vi "MainLoop2.vi"() -> ()   [LabVIEW 2021] (continued)
                                                                                                                                                                                                                                                                                                                                                                                                                                                                                                                                                                                                                                                                                                                                                                                                                                                                                                                                                                                                                                                                                                                                                                                                                                                                                                                                                                                                                                                                                                                                                                                                                                                                                                                                                                                                                                                                                                                                                                                                                                                                                                                                                                                                                                                                                                                                                                                                                                                                                                                                                                                                                                                                                                                                                                                                                                                                                                                                                                                                                                                                                                                                                                                                                                                                                                                                                                                                                                                                                                                                                                                                                                                                                                                                                                                                                                                                                                                                                                                                                                                                                                                                                                                                                                                                                                                                                                                                                                                                                                                                                                                                                                                                                                                                                                                                                                                                                                                                                                                                                                                                                                                                                                                                                                                                                                                                                                                                                                                                                                                                                                                                                                                                                                                                                                                                                                                                                                                                                                                                                                                                                                                                                                                                                                                                                                                                                                                                                                                                                                                                                                                                                                                                                                                                                                                                                                                                                                                                                                                                                                                                                                                                                                                                                                                                                                                                                                                                                                                                                                                                                                                                                                                                                                                                                                                                                                                                                                                                                                                                                                                                                                                                                                                                                                                                                                                                                                                                                                                                                                                                                                                                                                                                                                                                                                                                                                                                                                                                                                                                                                                                                                                                                                                                                                                                                                                                                                                                                                                                                                                                                                                                                                                                                                                                                                                                                                                                                                                                                                                                                                                                                                                                                                                                                                                                                                                                                                                                                                                                                                                                                                                                                                                                                                                                                                                                                                                                                                                                                                                                                                                                                                                                                                                                                                                                                                                                                                                                                                                                                                                                                                                                                                                                                                                                                                                                                                                                                                                                                                                                                                                                                                                                                                                                                                                                                                                                                                                                                                                                                                                                                                                                                                                                                                                                                                                                                                                                                                                                                                                                                                                                                                                                                                                                                                                                                                                                                                                                                                                                                                                                                                                                                                                                                                                                                                                                                                                                                                                                                                                                                                                                                                                                                                                                                                                                                                                                                                                                                                                                                                                                                                                                                                                                                                                                                                                                                                                                                                                                                                                                                                                                                                                                                                                                                                                                                                                                                                                                                                                                                                                                                                                                                                                                                                                                                                                                                                                                                                                                                                                                                                                                                                                                                                                                                                                                                                                                                                                                                                                                                                                                                                                                                                                                                                                                                                                                                                                                                                                                                                                                                                                                                                                                                                                                                                                                                                                                                                                                                                                                                                                                                                                                                                                                                                                                                                                                                                                                                                                                                                                                                                                                                                                                                                                                                                                                                                                                                                                                                                                                                                                                                                                                                                                                 256670997", "DINNER TIME", "0", "120", "0", "0", "0"], ["15/06/2022", "17:53:34", "256672767", "1 pellets delivered total", "0", "120", "0", "0", "0"], ["15/06/2022", "17:53:34", "256673260", "1 pellets delivered total", "0", "120", "1", "0", "0"], ["15/06/2022", "17:53:47", "256686605", "MIDDLE BEAM BREAK", "0", "201", "0", "0", "0"], ["15/06/2022", "17:53:48", "256686629", "Condition: m - 201", "0", "201", "0", "0", "0"], ["15/06/2022", "17:53:49", "256688396", "Nest beam break", "0", "201", "0", "0", "0"], ["15/06/2022", "17:53:53", "256692528", "4127 ms in nest", "0", "201", "0", "0", "0"], ["15/06/2022", "17:53:53", "256692552", "Nest beam break", "0", "201", "0", "0", "0"], ["15/06/2022", "17:53:56", "256694657", "SOCIAL TIME", "0", "201", "0", "0", "0"], ["15/06/2022", "17:53:59", "256697678", "SOCIAL TIME", "0", "201", "0", "0", "3009"], ["15/06/2022", "17:53:59", "256697702", "3009 ms social time", "0", "201", "0", "0", "3009"], ["15/06/2022", "17:54:00", "256699281", "MIDDLE BEAM BREAK", "0", "201", "0", "0", "0"], ["15/06/2022", "17:54:00", "256699306", "Condition: m - 201", "0", "201", "0", "0", "0"], ["15/06/2022", "17:54:05", "256704099", "DINNER TIME", "0", "201", "0", "0", "0"], ["15/06/2022", "17:54:06", "                                                                                                                                                                                                                                                                                                                                                                                                                                                                                                                                                                                                                                                                                                                                                                                                                                                                                                                                                                                                                                                              256705543", "Inter-pellet_interval", "0", "201", "0", "0", "0"], ["15/06/2022", "17:54:17", "                                                                                                                                                                                                                                                                                                                                                                                                                                                                                                                                                                                                                                                                                                                                                                                                                                                                                                                                                                                                                                                                                                                                                                                                                                                                                                                                                                                                                                                                                                                                                                                                                                                                                                                                                                                                                                                                                                                                                                                                                                                                                                                                                                                                                                                                                                                                                                                                                                                                                                                                                                                                                                                                                                                                                                                                                                                                                                                                                                                                                                                                                                                                                                                                                                                                                                                                                                                                                                                                                                                                                                                                                                                                                                                                                                                                                                                                                                                                                                                                                                                                                                                                                                                                                                                                                                                                                                                                                                                                                                                                                                                                                                                                                                                                                                                                                                                                                                                                                                                                                                                                                                                                                                                                                                                                                                                                                                                                                                                                                                                                                                                                                                                                                                                                                                                                                                                                                                                                                                                                                                                                                                                                                                                                                                                                                                                                                                                                                                                                                                                                                                                                                                                                                                                                                                                                                                                                                                                                                                                                                                                                                                                                                                                                                                                                                                                                                                                                                                                                                                                                                                                                                                                                                                                                                                                                                                                                                                                                                                                                                                                                                                                                                                                                                                                                                                                                                                                                                                                                                                                                                                                                                                                                                                                                                                                                                                                                                                                                                                                                                                                                                                                                                                                                                                                                                                                                                                                                                                                                                                                                                                                                                                                                                                                                                                                                                                                                                                                                                                                                                                                                                                                                                                                                                                                                                                                                                                                                                                                                                                                                                                                                                                                                                                                                                                                                                                                                                                                                                                                                                                                                                                                                                                                                                                                                                                                                                                                                                                                                                                                                                                                                                                          256715699", "3 pellets delivered total", "0", "201", "0", "0", "0"], ["15/06/2022", "17:54:17", "                                                                                                                                                                                                                                                                                                                                                                                                                                                                                                                                                                                                                                                                                                                                                                                                                                                                                                                                                                                                                                                                                                                                                                                                                                                                                                                                                                                                                                                                                                                                                                                                                                                                                                                                                                                                                                                                                                                                                                                                                                                                                                                                                                                                                                                                                                                                                                                                                                                                                                                                                                                                                                                                                                                                                                                                                                                                                                                                                                                                                                                                                                                                                                                                                                                                                                                                                                                                                                                                                                                                                                                                                                                                                                                                                                                                                                                                                                                                                                                                                                                                                                                                                                                                                                                                                                                                                                                                                                                                                                                                                                                                                                                                                                                                                                                                                                                                                                                                                                                                                                                                                                                                                                                                                                                                                                                                                                                                                                                                                                                                                                                                                                                                                                                                                                                                                                                                                                                                                                                                                                                                                                                                                                                                                                                                                                                                                                                                                                                                                                                                                                                                                                                                                                                                                                                                                                                                                                                                                                                                                                                                                                                                                                                                                                                                                                                                                                                                                                                                                                                                                                                                                                                                                                                                                                                                                                                                                                                                                                                                                                                                                                                                                                                                                                                                                                                                                                                                                                                                                                                                                                                                                                                                                                                                                                                                                                                                                                                                                                                                                                                                                                                                                                                                                                                                                                                                                                                                                                                                                                                                                                                                                                                                                                                                                                                                                                                                                                                                                                                                                                                                                                                                                                                                                                                                                                                                                                                                                                                                                                                                                                                                                                                                                                                                                                                                                                                                                                                                                                                                                                                                                                                                                                                                                                                                                                                                                                                                                                                                                                                                                                                                                                                                                                                                                                                                                                                                                                                                                                                                                                                                                                                              256716167", "3 pellets delivered total", "0", "201", "3", "0", "0"], ["15/06/2022", "17:54:50", "256749394", "3 pellets delivered total", "0", "120", "0", "0", "0"], ["15/06/2022", "17:54:50", "256749419", "Condition: j - 120", "0", "120", "0", "0", "0"], ["15/06/2022", "17:54:52", "256750710", "Nest beam break", "0", "120", "0", "0", "0"], ["15/06/2022", "18:19:22", "                                                                                                                                                                                                                                                                                                                                                                                                                                                                                                                                                                                                                                                                                                                                                                                                                                                                                                                                                                                                                                                                                                                                                                                                                                                                                                                                                                                                                                                                                                                                                                                                                                                                                                                                                                                                                                                                                                                                                                                                                                                                                                                                                                                                                                                                                                                                                                                                                                                                                                                                                                                                                                                                                                                                                                                                                                                                                                                                                                                                                                                                                                                                                                                                                                                                                                                                                                                                                                                                                                                                                                                                                                                                                                                                                                                                                                                                                                                                                                                                                                                                                                                                                                                                                                                                                                                                                                                                                                                                                                                                                                                                                                                                                                                                                                                                                                                                                                                                                                                                                                                                                                                                                                                                                                                                                                                                                                                                                                                                                                                                                                                                                                                                                                                                                                                                                                                                                                                                                                                                                                                                                                                                                                                                                                                                                                                                                                                                                                                                                                                                                                                                                                                                                                                                                                                                                                                                                                                                                                                                                                                                                                                                                                                                                                                                                                                                                                                                                                                                                                                                                                                                                                                                                                                                                                                                                                                                                                                                                                                                                                                                                                                                                                                                                                                                                                                                                                                                                                                                                                                                                                                                                                                                                                                                                                                                                                                                                                                                                                                                                                                                                                                                                                                                                                                                                                                                                                                                                                                                                                                                                                                                                                                                                                                                                                                                                                                                                                                                                                                              258221447", "1469059 ms in nest", "1469059", "120", "0", "0", "0"]]
  in  "Save event file?":bool=TRUE
  in  "file path (dialog if empty)":path=path "C:/Data/av_maze/cohort1/mouseX_202206XXtxt"
  # "Social\n\nWater\n\nFood\n\nMiddle 1\n\nMiddle 2\n\nHome cage"
  # "Low (0)     Medium (1)    High(2)"
  # "Pellets \n\nWater drops\n\nSocial time (ms)"
  # "This should stay at 1"
  # "Social                Water                  Food               Middle            Middle 2       Home cage"
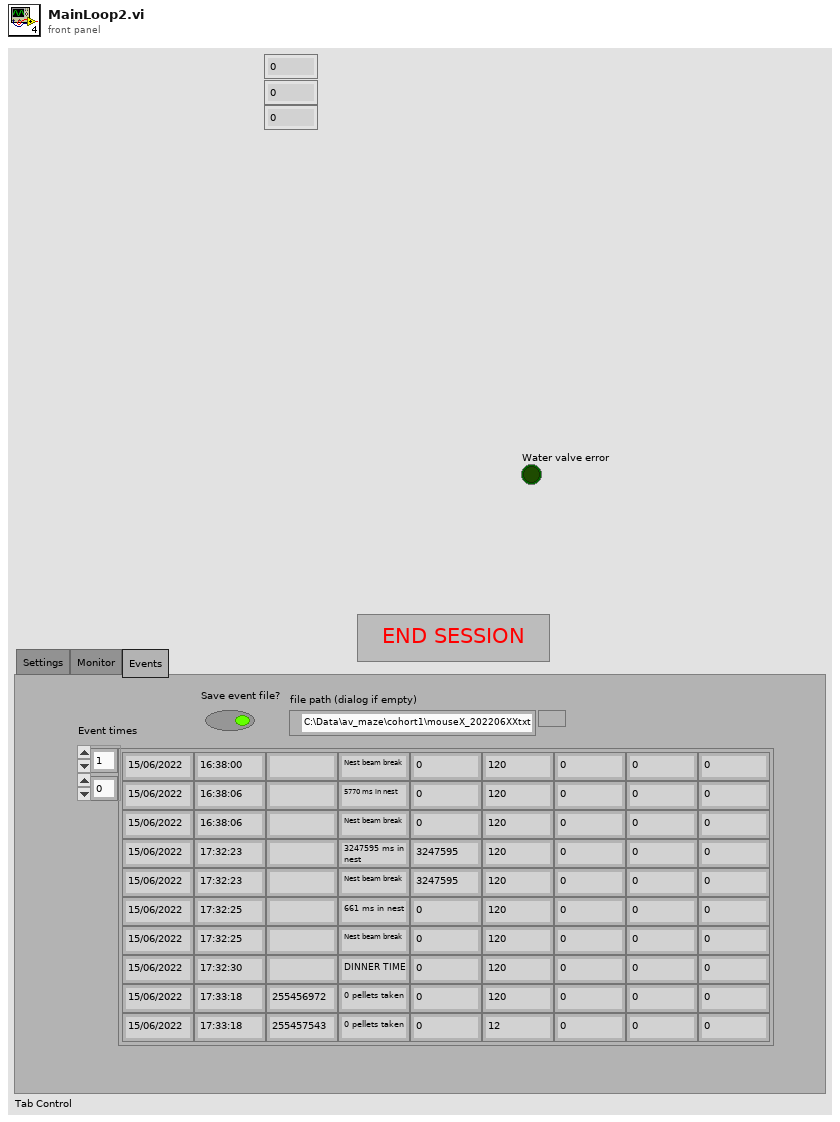
[diagram p1: front panel]
types:
  T1 = enum32{"All drives change and different", "One drive changes", "All drives same, but change"}
  T2 = typedef "XDNodeRunTimeDep.lvlib/timing_clust.ctl" = cluster{"Expected End [f-1]":u64, "Actual End [f-1]":u64, "Finished Late? [f-1]":bool, "Expected End [i-1]":u64, "Actual End [i-1]":u64, "Finished Late? [i-1]":bool, "Expected Start [i]":u64, "Actual Start [i]":u64, "Expected Start [f]":u64, "Actual Start [f]":u64, "Source Name":string, "Structure Name":string, "Period":i64, "Deadline":i64, "Offset":i64, "Start":i64, "Priority":i32, "Timeout":i32, "Mode":T3, "Wakeup Reason":T4, "Error":errorcluster, "Source Type":string, "Secondary Source Type":string, "Global End Time":u64, "Global Start Time":u64, "Frame Duration":u64, "Iteration Duration":u64, "Assigned CPU":i32, "I/O Scan Engine Mode":u32}
  T3 = typedef "XDNodeRunTimeDep.lvlib/nitl_modes.ctl" = enum32{"No Change", "Process missed periods, maintain original phase", "Discard missed periods, maintain original phase", "Process missed periods, ignore original phase", "Discard missed periods, ignore original phase"}
  T4 = typedef "XDNodeRunTimeDep.lvlib/wakeup.ctl" = enum32{"Normal", "Aborted", "Asynchronous wakeup", "Timing source error", "Timed loop error", "Timeout"}
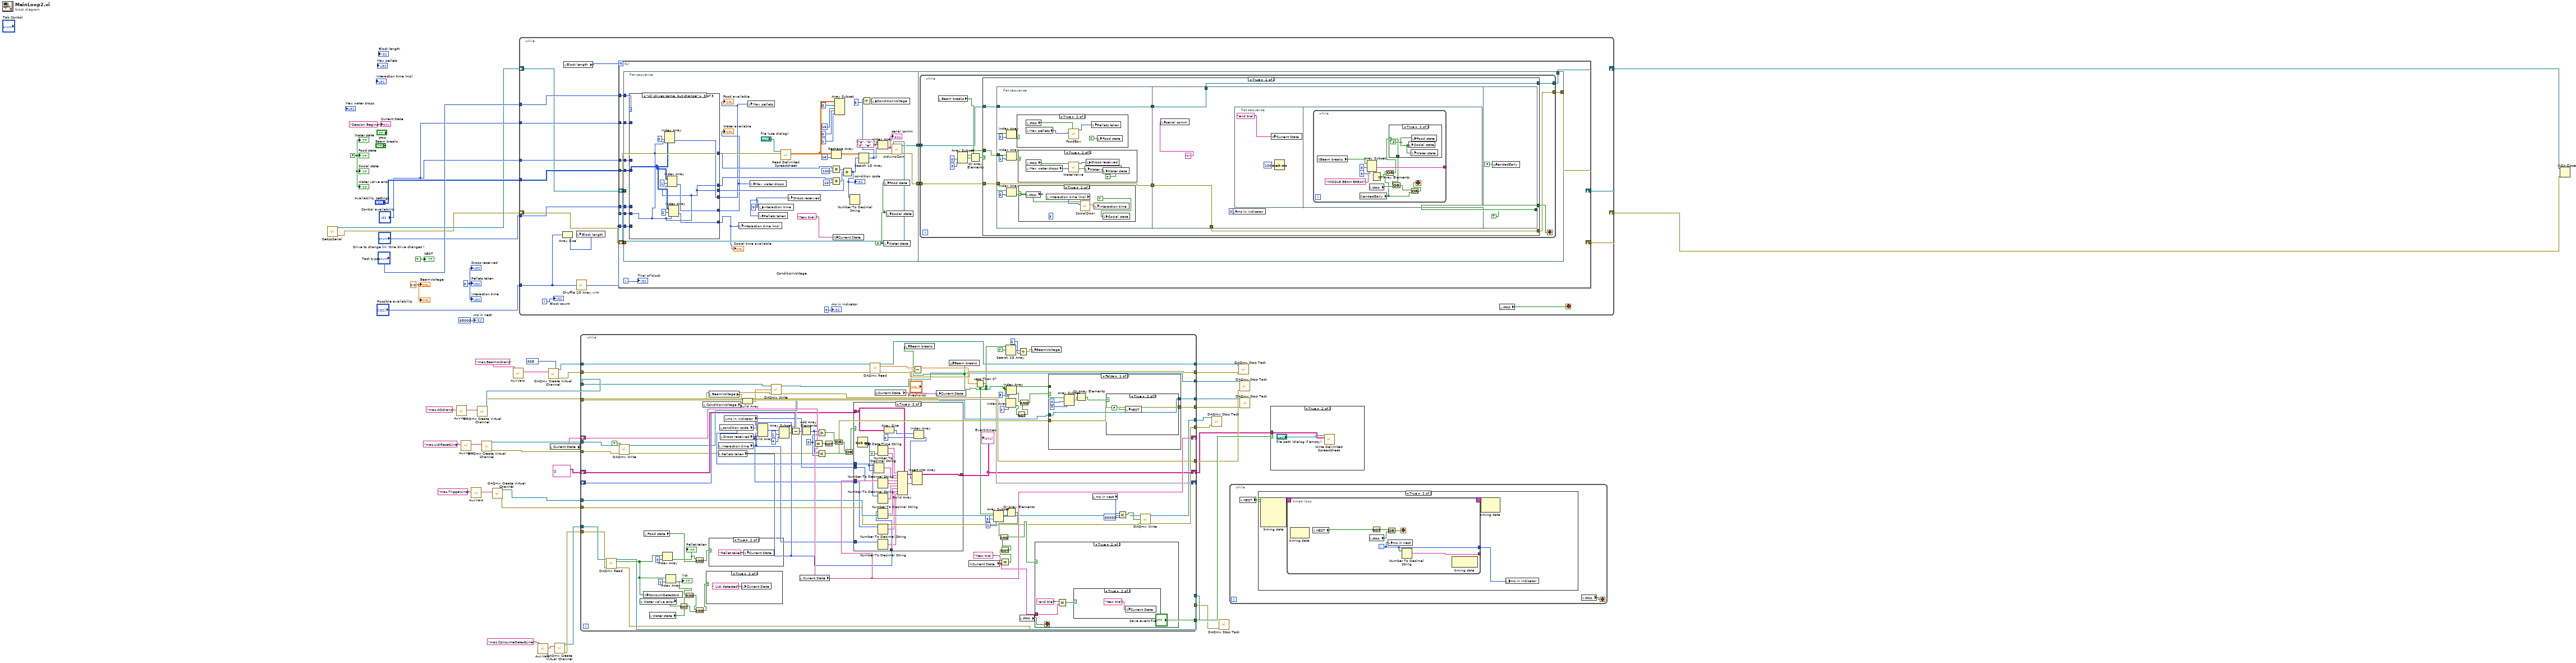
[diagram p0: block diagram]
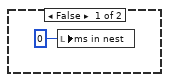
[diagram p2: hidden frame]
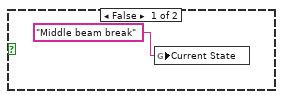
[diagram p7: hidden frame]
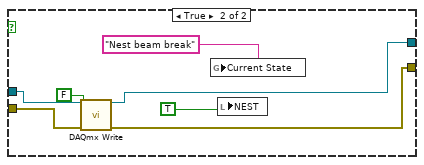
[diagram p9: hidden frame]
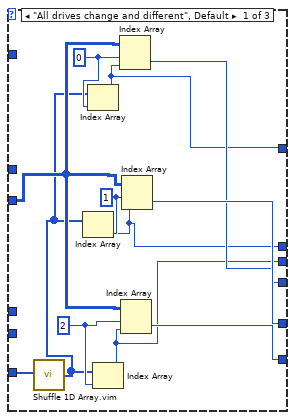
[diagram p11: hidden frame]
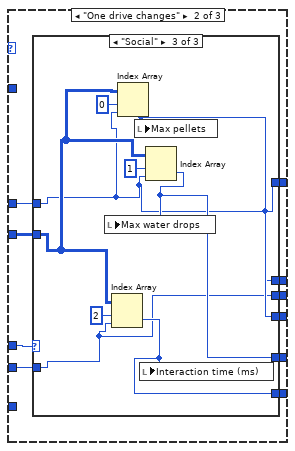
[diagram p12: hidden frame]
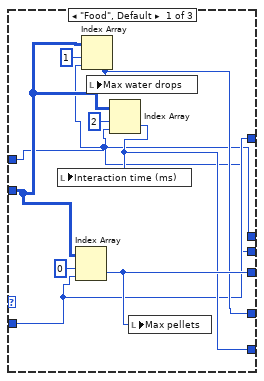
[diagram p13: hidden frame]
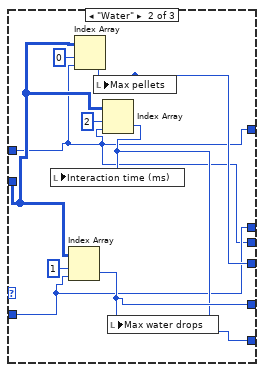
[diagram p14: hidden frame]
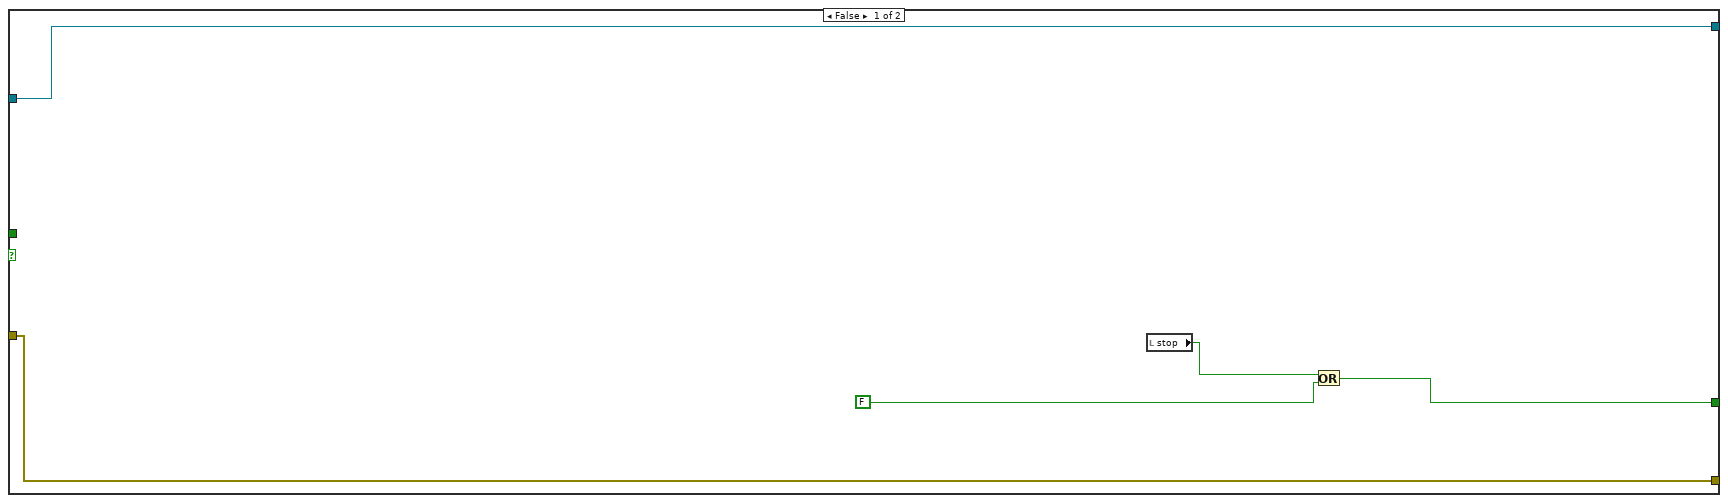
[diagram p15: hidden frame]
diagram:
  w13 = FALSE ("Water state")
  w22 = u32 0 ("Pellets taken")
  w33 = 0.0 ("BeamVoltage")
  w38 = 10083 items=["Default"=-1, "RSE"=10083, "NRSE"=10078, "Differential"=10106, "Pseudodifferential"=12529] ("input terminal configuration")
  n1 = call "SetUpSerial.vi"() -> ("error out"=w25:errorcluster, "VISA resource name out"=w40:refnum<visa-resource-name>)  [unwired: 10 in]
  n2 = call "AuxVars.vi"("key"="maz.AOchans") -> ("value"=w29:string)  [unwired: 9 in, 1 out]
  n3 = call "AuxVars.vi"("key"="maz.LickResetLine") -> ("value"=w12:string)  [unwired: 9 in, 1 out]
  n4 = call "AuxVars.vi"("key"="maz.TriggerLine") -> ("value"=w6:string)  [unwired: 9 in, 1 out]
  n5 = call-poly <vilib>:"DAQmx Create Virtual Channel.vi"("physical channels"=w29) -> ("task out"=w35:refnum<k21>, "error out"=w34:errorcluster)  [unwired: 13 in]
  n6 = call-poly <vilib>:"DAQmx Create Virtual Channel.vi"("lines"=w12) -> ("task out"=w10:refnum<k21>, "error out"=w9:errorcluster)  [unwired: 13 in]
  n7 = call-poly <vilib>:"DAQmx Create Virtual Channel.vi"("lines"=w6) -> ("task out"=w4:refnum<k21>, "error out"=w3:errorcluster)  [unwired: 13 in]
  n8 = call "AuxVars.vi"("key"="maz.BeamAIchans") -> ("value"=w27:string)  [unwired: 9 in, 1 out]
  n9 = while {
    tunnel: "Task type" -> [w66]
    tunnel: "Drive to change (in 'One drive changes')" -> [w65]
    tunnel: "Possible availability" -> [w60]
    tunnel: "Availability settings" -> [w64]
    tunnel: "Control availability" -> [w63]
    tunnel: "Control availability" -> [w62]
    shift-right: [w53] -> w26
    shift-left: w40 -> [w55]
    shift-right: [w52] -> w39
    shift-left: w25 -> [w54]
    i -> [w58]
    stop <- w56 stop-if-true
    n10 = Array Size(array=w60) -> (size(s)=w59:i32)
    n11 = local read "Block length"() -> (w61:i32)
    n12 = local write "Block length"(w59) -> ()
    n13 = call "Shuffle 1D Array.vim"("array"=w60) -> ("shuffled array"=w57:i32[])  [unwired: 4 in]
    n14 = for {
      N: w61 -> [_]
      tunnel: w66 -> [w80]
      tunnel: w65 -> [w79]
      tunnel: w57 -> [w78] mode=indexing
      tunnel: w64 -> [w77]
      tunnel: w63 -> [w76]
      tunnel: w62 -> [w75]
      tunnel: w57 -> [w73]
      shift-right: [w68] -> w53
      shift-left: w55 -> [w72]
      shift-right: [w67] -> w52
      shift-left: w54 -> [w71]
      i -> [w74]
      n15 = flat-sequence {
        tunnel: w80 -> [w118]
        tunnel: w79 -> [w117]
        tunnel: w78 -> [w116]
        tunnel: w77 -> [w115]
        tunnel: w76 -> [w114]
        tunnel: w75 -> [w113]
        tunnel: w73 -> [w112]
        tunnel: w72 -> [w93]
        tunnel: w71 -> [w92]
        tunnel: [w82] -> w70
        tunnel: [w81] -> w69
        tunnel: w70 -> [w179]
        tunnel: w69 -> [w178]
        tunnel: [w177] -> w68
        tunnel: [w176] -> w67
        frame #0 {
          w84 = FALSE ("Social state")
          w85 = u32 0 ("interaction time")
          n16 = case shown="\"All drives same, but change\"" w118 {
            tunnel: w117 -> [_ w140 _]
            tunnel: w116 -> [_ w139 w168]
            tunnel: w115 -> [w130 w138 w172]
            tunnel: w114 -> [_ _ _]
            tunnel: w113 -> [_ w137 _]
            tunnel: [w122 w136 w171] -> w90
            tunnel: [w123 w135 w170] -> w89
            tunnel: [w127 w134 w169] -> w91
            tunnel: w112 -> [w129 _ _]
            tunnel: [w121 w133 w168] -> w109
            tunnel: [w120 w132 w168] -> w108
            tunnel: [w119 w131 w168] -> w107
            frame "All drives change and different", Default {
              w126 = 0 ("index")
              w125 = 1 ("index")
              w128 = 2 ("index")
              n17 = call "Shuffle 1D Array.vim"("array"=w129) -> ("shuffled array"=w124:i32[])  [unwired: 4 in]
              n18 = Index Array(array=w124, index=w125) -> (element=w120:i32)
              n19 = Index Array(array=w124, index=w126) -> (element=w121:i32)
              n20 = Index Array(array=w124, index=w128) -> (element=w119:i32)
              n21 = Index Array(array=w130, index (row)=w126, index (col)=w121) -> (element=w122:i32)
              n22 = Index Array(array=w130, index (row)=w128, index (col)=w119) -> (element=w127:i32)
              n23 = Index Array(array=w130, index (row)=w125, index (col)=w120) -> (element=w123:i32)
            }
            frame "One drive changes" {
              n24 = case shown="\"Social\"" w140 {
                tunnel: w139 -> [w142 w151 w159]
                tunnel: w138 -> [w146 w155 w164]
                tunnel: w137 -> [w141 w150 w160]
                tunnel: [w145 w154 w161] -> w136
                tunnel: [w144 w153 w163] -> w135
                tunnel: [w143 w152 w162] -> w134
                tunnel: [w142 w150 w160] -> w133
                tunnel: [w141 w151 w160] -> w132
                tunnel: [w141 w150 w159] -> w131
                frame "Food", Default {
                  n25 = Index Array(array=w146, index (row)=0 ("index"), index (col)=w142) -> (element=w145:i32)
                  n26 = Index Array(array=w146, index (row)=1, index (col)=w141) -> (element=w144:i32)
                  n27 = local write "Max water drops"(w144) -> ()
                  n28 = Index Array(array=w146, index (row)=2 ("disabled index (row)"), index (col)=w141) -> (element=w143:i32)
                  n29 = local write "Interaction time (ms)"(w143) -> ()
                  n30 = local write "Max pellets"(w145) -> ()
                }
                frame "Water" {
                  n31 = Index Array(array=w155, index (row)=1 ("index"), index (col)=w151) -> (element=w153:i32)
                  n32 = Index Array(array=w155, index (row)=0, index (col)=w150) -> (element=w154:i32)
                  n33 = local write "Max pellets"(w154) -> ()
                  n34 = Index Array(array=w155, index (row)=2 ("disabled index (row)"), index (col)=w150) -> (element=w152:i32)
                  n35 = local write "Interaction time (ms)"(w152) -> ()
                  n36 = local write "Max water drops"(w153) -> ()
                }
                frame "Social" {
                  n37 = Index Array(array=w164, index (row)=2 ("index"), index (col)=w159) -> (element=w162:i32)
                  n38 = Index Array(array=w164, index (row)=0, index (col)=w160) -> (element=w161:i32)
                  n39 = local write "Max pellets"(w161) -> ()
                  n40 = local write "Interaction time (ms)"(w162) -> ()
                  n41 = Index Array(array=w164, index (row)=1 ("disabled index (row)"), index (col)=w160) -> (element=w163:i32)
                  n42 = local write "Max water drops"(w163) -> ()
                }
              }
            }
            frame "All drives same, but change" {
              n43 = Index Array(array=w172, index (row)=0, index (col)=w168) -> (element=w171:i32)
              n44 = Index Array(array=w172, index (row)=1, index (col)=w168) -> (element=w170:i32)
              n45 = Index Array(array=w172, index (row)=2, index (col)=w168) -> (element=w169:i32)
            }
          }
          "Food available" <- w90
          "Water available" <- w89
          "Social time available" <- w91
          n46 = local write "Interaction time (ms)"(w91) -> ()
          n47 = local write "Max pellets"(w90) -> ()
          n48 = local write "Max water drops"(w89) -> ()
          n49 = local write "interaction time"(w85) -> ()
          n50 = local write "Pellets taken"(w85) -> ()
          n51 = call-poly <vilib>:"Read Delimited Spreadsheet.vi"("file path (dialog if empty)"="file (use dialog)") -> ("all rows"=w99:dbl[][])  [unwired: 9 in, 5 out]
          n52 = local write "Drops received"(w85) -> ()
          n53 = Reshape Array(w99, 16 ("dimension size")) -> (w98:dbl[])
          n54 = Multiply(x=w109, y=100) -> (x*y=w105:i32)
          n55 = Multiply(x=w108, y=10) -> (x*y=w106:i32)
          n56 = global write "GlobalSTATE.vi" "Current State"("New trial " ("string")) -> ()
          n57 = Array Subset(array=w99, index (row)=0 ("index"), length (row)=16 ("length"), index (col)=0 ("index"), length (col)=1 ("length")) -> ()  [unwired: 1 out]
          n58 = Compound Arithmetic op=ADD(w105, w106, w107) -> (w94:i32)
          "condition code" <- w94
          n59 = Number To Decimal String(number=w94) -> ()  [unwired: 1 in, 1 out]
          n60 = Search 1D Array(1D array=w98, element=w94) -> (index of element=w87:i32)  [unwired: 1 in]
          n61 = Divide(x=w87, y=5) -> (x/y=w88:dbl)
          n62 = local write "ConditionVoltage"(w88) -> ()
          n63 = Index Array(array=string[] ["a", "b", "c", "d", "e", "f", "g", "h", "i", "j", "k", "l", "m", "n", "o"], index=w87) -> (element=w95:string)
          "serial comm" <- w95
          n64 = local write "Water state"(w84) -> ()
          n65 = local write "Food state"(w84) -> ()
          n66 = local write "Social state"(w84) -> ()
          n67 = call "ArduinoCom.vi"("error out"=w92, "write buffer"=w95, "VISA resource name out"=w93) -> ("error out 2"=w81:errorcluster, "VISA resource name out 2"=w82:refnum<visa-resource-name>)  [unwired: 7 in]
        }
        frame #1 {
          n68 = while {
            tunnel: w179 -> [w183]
            tunnel: w178 -> [w182]
            tunnel: [w181] -> w177
            tunnel: [w180] -> w176
            stop <- w184 stop-if-true
            n69 = local read "Beam breaks"() -> (w185:bool[])
            n70 = Array Subset(array=w185, index=0, length=3) -> (w188:bool[])
            n71 = Or Array Elements(Boolean array=w188) -> (logical OR=w189:bool)
            n72 = case shown="True" w189 {
              tunnel: w185 -> [_ w202]
              tunnel: [w192 w201] -> w184
              tunnel: w183 -> [w191 w199]
              tunnel: w182 -> [w190 w197]
              tunnel: [w191 w196] -> w181
              tunnel: [w190 w195] -> w180
              frame False {
                n73 = local read "stop"() -> (w193:bool)
                n74 = Or(x=w193, y=FALSE ("stop")) -> (x .or. y?=w192:bool)
              }
              frame True {
                n75 = flat-sequence {
                  tunnel: w202 -> [w205]
                  tunnel: [w204] -> w200
                  tunnel: w199 -> [w204]
                  tunnel: [w203] -> w198
                  tunnel: w197 -> [w203]
                  tunnel: w200 -> [w227]
                  tunnel: w198 -> [w226]
                  tunnel: [w227] -> w196
                  tunnel: [w226] -> w195
                  tunnel: [TRUE ("stop")] -> w201
                  frame #0 {
                    n76 = Index Array(array=w205, index=2) -> (element=w210:bool)
                    n77 = Index Array(array=w205, index=1) -> (element=w206:bool)
                    n78 = Index Array(array=w205, index=0) -> (element=w208:bool)
                    n79 = case shown="True" w210 {
                      frame False {
                      }
                      frame True {
                        n80 = local read "stop"() -> (w223:bool)
                        n81 = local read "Max pellets"() -> (w224:u32)
                        n82 = call "FoodBox.vi"("STOP"=w223, "Max pellets"=w224) -> ("Pellets taken"=w222:i32)  [unwired: 8 in, 1 out]
                        n83 = local write "Pellets taken"(w222) -> ()
                        n84 = local write "Food state"(TRUE ("Food state")) -> ()
                      }
                    }
                    n85 = case shown="True" w206 {
                      frame False {
                      }
                      frame True {
                        n86 = local read "stop"() -> (w215:bool)
                        n87 = local read "Max water drops"() -> (w216:u32)
                        n88 = call "WaterValve.vi"("Max pulses"=w216, "STOP"=w215) -> ("Error"=w212:bool, "Number pulses"=w214:u32)  [unwired: 8 in]
                        n89 = local write "Water valve error"(w212) -> ()
                        n90 = local write "Drops received"(w214) -> ()
                        n91 = local write "Water state"(TRUE ("Water state")) -> ()
                      }
                    }
                    n92 = case shown="True" w208 {
                      frame False {
                      }
                      frame True {
                        (unwired) 3 ("index")
                        n93 = local read "stop"() -> (w219:bool)
                        n94 = local read "Interaction time (ms)"() -> (w220:u32)
                        n95 = call "SocialDoor.vi"("Interaction time"=w220, "STOP"=w219) -> ("Time spent"=w218:dbl)  [unwired: 9 in]
                        n96 = local write "interaction time"(w218) -> ()
                        n97 = local write "Social state"(TRUE ("Water state")) -> ()
                      }
                    }
                  }
                  frame #1 {
                    n98 = local write "serial comm"("h" ("write buffer")) -> ()
                    n99 = local write "ms in indicator"(0 ("ms in nest")) -> ()
                    n100 = flat-sequence {
                      frame #0 {
                        n101 = global write "GlobalSTATE.vi" "Current State"("end trial " ("string")) -> ()
                        n102 = Wait (ms)(milliseconds to wait=u32 100) -> ()  [unwired: 1 out]
                      }
                      frame #1 {
                        n103 = while {
                          tunnel: ["MIDDLE BEAM BREAK" ("Current State")] -> _
                          stop <- w234 stop-if-true
                          n104 = global read "Global_BeamBreaks.vi" "Beam breaks"() -> (w238:bool[])
                          n105 = global read "EndEarly.vi" "endedEarly"() -> (w232:bool)
                          n106 = Array Subset(array=w238, index=3, length=3) -> (w237:bool[])
                          n107 = local read "stop"() -> (w241:bool)
                          n108 = Or Array Elements(Boolean array=w237) -> (logical OR=w233:bool)
                          n109 = Or(x=w232, y=w233) -> (x .or. y?=w231:bool)
                          n110 = case shown="True" w231 {
                            selector: w231 -> [w243 w244]
                            tunnel: [w243 w244] -> w236
                            frame False {
                            }
                            frame True {
                              w245 = FALSE ("Social state")
                              n111 = local write "Social state"(w245) -> ()
                              n112 = local write "Water state"(w245) -> ()
                              n113 = local write "Food state"(w245) -> ()
                            }
                          }
                          n114 = Or(x=w236, y=w241) -> (x .or. y?=w235:bool)
                          n115 = Or(x=w235, y=w232) -> (x .or. y?=w234:bool)
                        }
                      }
                    }
                  }
                  frame #2 {
                    n116 = global write "EndEarly.vi" "endedEarly"(FALSE ("endedEarly")) -> ()
                  }
                }
              }
            }
          }
        }
      }
      "Trial of block" <- w74
    }
    n117 = local read "stop"() -> (w56:bool)
    "Block count" <- w58
  }
  n118 = call "AuxVars.vi"("key"="maz.ConsumeDetectLine") -> ("value"=w18:string)  [unwired: 9 in, 1 out]
  n119 = call-poly <vilib>:"DAQmx Create Virtual Channel.vi"("input terminal configuration"=w38, "physical channels"=w27) -> ("task out"=w51:refnum<k21>, "error out"=w50:errorcluster)  [unwired: 12 in]
  n120 = local read "Current State"() -> (w41:string)
  n121 = call-poly <vilib>:"DAQmx Create Virtual Channel.vi"("lines"=w18) -> ("task out"=w17:refnum<k21>, "error out"=w16:errorcluster)  [unwired: 13 in]
  n122 = while {
    tunnel: w51 -> [w337]
    tunnel: w50 -> [w336]
    tunnel: [w335] -> w49
    tunnel: [w334] -> w48
    shift-right: [w331] -> _
    shift-left: w41 -> [w330]
    tunnel: ["Save event file?"] -> w37
    tunnel: w35 -> [w323]
    tunnel: w34 -> [w322]
    tunnel: [w314] -> w32
    tunnel: [w313] -> w31
    shift-right: [w307] -> _
    shift-left: _ -> [w312]
    shift-right: [w299] -> w24
    shift-left: string[][] [] -> [w298]
    tunnel: w17 -> [w289]
    tunnel: w16 -> [w288]
    tunnel: [w282] -> w15
    tunnel: [w281] -> w14
    tunnel: w10 -> [w261]
    tunnel: w9 -> [w260]
    tunnel: [w256] -> w8
    tunnel: [w255] -> w7
    tunnel: w4 -> [w251]
    tunnel: w3 -> [w250]
    tunnel: [w249] -> w2
    tunnel: [w248] -> w1
    stop <- w333 stop-if-true
    w304 = u32 0 ("y")
    n123 = call-poly <vilib>:"DAQmx Read.vi"("task/channels in"=w289, "error in"=w288) -> ("task out"=w282:refnum<k21>, "data"=w285:bool[], "error out"=w281:errorcluster)  [unwired: 11 in]
    n124 = call-poly <vilib>:"DAQmx Write.vi"("task/channels in"=w261, "data"=TRUE, "error in"=w260) -> ("task out"=w258:refnum<k21>, "error out"=w257:errorcluster)  [unwired: 10 in, 1 out]
    n125 = local read "Water valve error"() -> (w277:bool)
    n126 = global write "Global_BeamBreaks.vi" "ConsumDetectors"(w285) -> ()
    n127 = local read "Food state"() -> (w278:bool)
    n128 = local read "Water state"() -> (w283:bool)
    n129 = Index Array(array=w285, index=0) -> (element=w279:bool)
    "Pellet taken" <- w279
    n130 = Index Array(array=w285, index=1) -> (element=w284:bool)
    "lick" <- w284
    n131 = Not(x=w277) -> (.not. x?=w276:bool)
    n132 = And(x=w284, y=w283) -> (x .and. y?=w275:bool)
    n133 = And(x=w279, y=w278) -> (x .and. y?=w280:bool)
    n134 = And(x=w275, y=w276) -> (x .and. y?=w274:bool)
    n135 = local read "ConditionVoltage"() -> (w316:dbl)
    n136 = case shown="True" w274 {
      frame False {
      }
      frame True {
        n137 = local write "Current State"(" Lick detected" ("Current State")) -> ()
      }
    }
    n138 = local read "BeamVoltage"() -> (w317:dbl)
    n139 = case shown="True" w280 {
      frame False {
      }
      frame True {
        n140 = local write "Current State"("Pellet taken" ("Current State")) -> ()
      }
    }
    n141 = local read "interaction time"() -> (w293:u32)
    n142 = local read "Pellets taken"() -> (w296:u32)
    n143 = local read "condition code"() -> (w297:i32)
    n144 = local read "Drops received"() -> (w295:u32)
    n145 = local read "ms in indicator"() -> (w294:i32)
    n146 = Build Array(w317, w316) -> (w315:dbl[])
    n147 = Build Array(w294, w297, w296, w295, w293) -> (w300:u32[])
    n148 = call-poly <vilib>:"DAQmx Write.vi"("task/channels in"=w323, "data"=w315, "error in"=w322) -> ("task out"=w314:refnum<k21>, "error out"=w313:errorcluster)  [unwired: 10 in, 1 out]
    n149 = Array Subset(array=w300, index=1, length=4) -> (w307:u32[])
    n150 = Subtract(x=w312, y=w307) -> (x-y=w306:u32[])
    n151 = local read "Current State"() -> (w331:string)
    n152 = Add Array Elements(numeric array=w306) -> (sum=w305:u32)
    n153 = Equal?(x=w330, y=w331) -> (x = y?=w332:bool)
    n154 = Greater?(x=w305, y=w304) -> (0:w310:bool)
    n155 = Less?(x=w305, y=w304) -> (x < y?=w302:bool)
    n156 = Not(x=w332) -> (.not. x?=w311:bool)
    n157 = Or(x=w310, y=w311) -> (x .or. y?=w303:bool)
    n158 = Or(x=w303, y=w302) -> (x .or. y?=w301:bool)
    n159 = case shown="True" w301 {
      tunnel: [w360 w375] -> w299
      tunnel: w331 -> [_ w377]
      tunnel: w298 -> [w360 w374]
      tunnel: w294 -> [_ w370]
      tunnel: w297 -> [_ w368]
      tunnel: w296 -> [_ w366]
      tunnel: w295 -> [_ w364]
      tunnel: w293 -> [_ w361]
      frame False {
      }
      frame True {
        n160 = Tick Count (ms)() -> (millisecond timer value=w381:u32)
        n161 = Number To Decimal String(number=w381, width (-)=w381) -> (decimal integer string=w378:string)
        n162 = Get Date/Time String(want seconds? (F)=TRUE) -> (date string=w380:string, time string=w379:string)  [unwired: 2 in]
        n163 = Number To Decimal String(number=w370) -> (decimal integer string=w369:string)  [unwired: 1 in]
        n164 = Number To Decimal String(number=w368) -> (decimal integer string=w367:string)  [unwired: 1 in]
        n165 = Number To Decimal String(number=w366) -> (decimal integer string=w365:string)  [unwired: 1 in]
        n166 = Number To Decimal String(number=w364) -> (decimal integer string=w363:string)  [unwired: 1 in]
        n167 = Number To Decimal String(number=w361) -> (decimal integer string=w362:string)  [unwired: 1 in]
        n168 = Array Size(array=w374) -> (size(s)=w373:i32[])
        n169 = Build Array(w380, w379, w378, w377, w369, w367, w365, w363, w362) -> (w376:string[])
        n170 = Index Array(array=w373, index=0) -> (element=w371:i32)
        n171 = Insert Into Array(array=w374, index (row)=w371, new element=w376) -> (w375:string[][])  [unwired: 1 in]
      }
    }
    "Event times" <- w299
    n172 = call-poly <vilib>:"DAQmx Read.vi"("task/channels in"=w337, "error in"=w336) -> ("task out"=w335:refnum<k21>, "data"=w327:dbl[], "error out"=w334:errorcluster)  [unwired: 11 in]
    n173 = global read "GlobalSTATE.vi" "Current State"() -> (w329:string)
    n174 = Subtract(x=w327, y="thresholds") -> (x-y=w328:dbl[])
    n175 = local write "Current State"(w329) -> ()
    n176 = global read "GlobalSTATE.vi" "Current State"() -> (w262:string)
    n177 = Less Than 0?(x=w328) -> (x < 0?=w272:bool[])
    n178 = local write "Beam breaks"(w272) -> ()
    n179 = global write "Global_BeamBreaks.vi" "Beam breaks"(w272) -> ()
    n180 = Array Subset(array=w272, index=3, length=2) -> (w290:bool[])
    n181 = Equal?(x="New trial " ("string"), y=w262) -> (x = y?=w266:bool)
    n182 = Not(x=w266) -> (.not. x?=w267:bool)
    n183 = Search 1D Array(1D array=w272, element=TRUE) -> (index of element=w321:i32)  [unwired: 1 in]
    n184 = Index Array(array=w272, index=4) -> (element=w271:bool)
    n185 = Or Array Elements(Boolean array=w290) -> (logical OR=w264:bool)
    n186 = And(x=w264, y=w267) -> (x .and. y?=w263:bool)
    n187 = Index Array(array=w272, index=5) -> (element=w269:bool)
    n188 = Not(x=w271) -> (.not. x?=w270:bool)
    n189 = Divide(x=w321, y=2) -> (x/y=w319:dbl)
    n190 = And(x=w269, y=w270) -> (x .and. y?=w268:bool)
    n191 = local read "stop"() -> (w333:bool)
    n192 = local write "BeamVoltage"(w319) -> ()
    n193 = case shown="True" w263 {
      tunnel: w262 -> [_ w341]
      frame False {
      }
      frame True {
        n194 = Equal?(x="end trial" ("string"), y=w341) -> (x = y?=w340:bool)
        n195 = case shown="True" w340 {
          frame False {
            n196 = global write "GlobalSTATE.vi" "Current State"("Middle beam break" ("Current State")) -> ()
          }
          frame True {
            n197 = global write "GlobalSTATE.vi" "Current State"("New trial" ("Current State")) -> ()
          }
        }
      }
    }
    n198 = case shown="False" w268 {
      tunnel: w272 -> [w351 _]
      tunnel: w258 -> [w346 w357]
      tunnel: w257 -> [w345 w356]
      tunnel: [w346 w354] -> w256
      tunnel: [w345 w353] -> w255
      frame False {
        n199 = Array Subset(array=w351, index=0, length=5) -> (w348:bool[])
        n200 = Or Array Elements(Boolean array=w348) -> (logical OR=w347:bool)
        n201 = case shown="True" w347 {
          frame False {
          }
          frame True {
            n202 = local write "NEST"(FALSE) -> ()
          }
        }
      }
      frame True {
        n203 = call-poly <vilib>:"DAQmx Write.vi"("task/channels in"=w357, "data"=FALSE, "error in"=w356) -> ("task out"=w354:refnum<k21>, "error out"=w353:errorcluster)  [unwired: 10 in, 1 out]
        n204 = global write "GlobalSTATE.vi" "Current State"("Nest beam break" ("Current State")) -> ()
        n205 = local write "NEST"(TRUE) -> ()
      }
    }
    n206 = local read "ms in nest"() -> (w254:i32)
    n207 = Less?(x=w254, y=u32 60000) -> (x < y?=w252:bool)
    n208 = call-poly <vilib>:"DAQmx Write.vi"("task/channels in"=w251, "data"=w252, "error in"=w250) -> ("task out"=w249:refnum<k21>, "error out"=w248:errorcluster)  [unwired: 10 in, 1 out]
  }
  n209 = call <vilib>:"DAQmx Stop Task.vi"("task/channels in"=w2, "error in"=w1) -> ()  [unwired: 12 in, 2 out]
  n210 = call <vilib>:"DAQmx Stop Task.vi"("task/channels in"=w15, "error in"=w14) -> ()  [unwired: 12 in, 2 out]
  n211 = while {
    stop <- w383 stop-if-true
    n212 = local read "NEST"() -> (w384:bool)
    n213 = case shown="True" w384 {
      frame False {
        n214 = local write "ms in nest"(0 ("ms in nest")) -> ()
      }
      frame True {
        n215 = node-c288() -> (w388:T2)  [unwired: 4 in]
        n216 = timed-loop {
          timing: w388 -> [_]
          timing-out: [_] -> w387
          tunnel: [w393] -> _
          tunnel: [w389] -> w386
          i -> [w389]
          stop <- w390 stop-if-true
          n217 = node-c288() -> ()  [unwired: 1 in, 1 out]
          n218 = local read "NEST"() -> (w394:bool)
          n219 = local read "stop"() -> (w391:bool)
          n220 = Not(x=w394) -> (.not. x?=w392:bool)
          n221 = Or(x=w392, y=w391) -> (x .or. y?=w390:bool)
          n222 = local write "ms in nest"(w389) -> ()
          n223 = Number To Decimal String(number=w389) -> (decimal integer string=w393:string)  [unwired: 1 in]
          n224 = node-c288() -> ()  [unwired: 1 in, 1 out]
        }
        n225 = node-c288(w387) -> ()  [unwired: 1 out]
        n226 = local write "ms in indicator"(w386) -> ()
      }
    }
    n227 = local read "stop"() -> (w383:bool)
  }
  n228 = call <vilib>:"DAQmx Stop Task.vi"("task/channels in"=w49, "error in"=w48) -> ()  [unwired: 12 in, 2 out]
  n229 = call <vilib>:"DAQmx Stop Task.vi"("task/channels in"=w32, "error in"=w31) -> ()  [unwired: 12 in, 2 out]
  n230 = call <vilib>:"DAQmx Stop Task.vi"("task/channels in"=w8, "error in"=w7) -> ()  [unwired: 12 in, 2 out]
  n231 = case shown="True" w37 {
    tunnel: w24 -> [_ w400]
    frame False {
    }
    frame True {
      n232 = call-poly <vilib>:"Write Delimited Spreadsheet.vi"("file path (dialog if empty)"="file path (dialog if empty)", "2D data"=w400) -> ()  [unwired: 12 in, 2 out]
    }
  }
  n233 = VISA Close(VISA resource name=w26, error in (no error)=w39) -> ()  [unwired: 1 out]
  "Current State" <- "Session Begins" ("Current State")
  "ms in nest" <- 65000 ("ms in nest")
  "NEST" <- TRUE ("NEST")
  "BeamVoltage" <- w33
  "ConditionVoltage" <- w33
  "interaction time" <- w22
  "Drops received" <- w22
  "Pellets taken" <- w22
  "ms in indicator" <- 0 ("ms in indicator")
  "Food state" <- w13
  "Social state" <- w13
  "Water state" <- w13
  "Water valve error" <- w13
